vi "MB Serial Master Query.vi"(4 "Timeout":u32=10000, 6 "Serial Parameters":T1 {"Slave Address" format="%.0x"}, 8 "error in (no error)":errorcluster, 10 "Modbus Command":T2={"Function Code"=1, "Starting Address"=0, "Quantity"=0, "Data"=[], "Discrete"=[], "Index of Tags"=[]} {"Function Code" items=["Read Coils"=1, "Read Discrete Inputs"=2, "Read Holding Registers"=3, "Read Input Registers"=4, "Write Single Coil"=5, "Write Single Register"=6, "Read Exception Status"=7, "Write Multiple Coils"=15, "Write Multiple Registers"=16]}, 11 "VISA resource name":refnum<visa-resource-name>) -> (0 "error out":errorcluster, 1 "Exception Code":u8 format="%.0x", 2 "Registers":cluster{"Registers":u16[], "Discrete":bool[]}, 3 "VISA resource name out":refnum<visa-resource-name>, 5 "Modbus Data Unit Out":T3={"Function Code"=1, "Data"=[]} {"Function Code" items=["Read Coils"=1, "Read Discrete Inputs"=2, "Read Holding Registers"=3, "Read Input Registers"=4, "Write Single Coil"=5, "Write Single Register"=6, "Read Exception Status"=7, "Write Multiple Coils"=15, "Write Multiple Registers"=16]; "Data" format="%.0x"}, 7 "read buffer":string)   [LabVIEW 2020, in "ModBus Serial Master.lvlib"]
uses:
  ModBus Serial Master.lvlib
  MB Modbus Data Unit.ctl
  DriverCommon/MB Modbus Command.ctl
  DriverCommon.lvlib
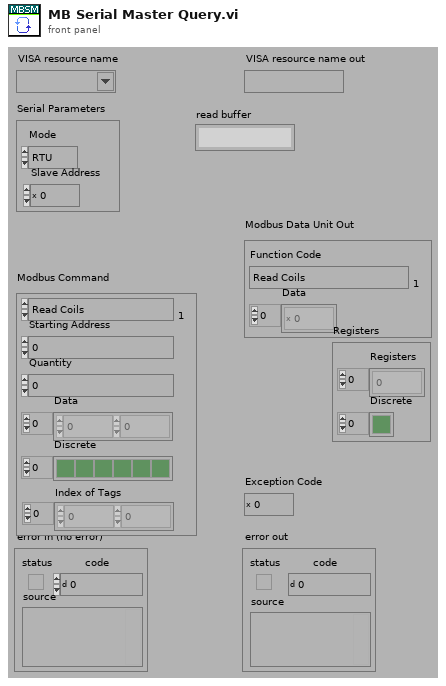
[diagram p1: front panel]
types:
  T1 = cluster{"Mode":enum16{"RTU", "ASCII"}, "Slave Address":u8}
  T2 = typedef "DriverCommon.lvlib/MB Modbus Command.ctl" = cluster{"Function Code":u8, "Starting Address":u16, "Quantity":u16, "Data":u16[], "Discrete":bool[], "Index of Tags":i32[]}
  T3 = typedef "ModBus Serial Master.lvlib/MB Modbus Data Unit.ctl" = cluster{"Function Code":u8, "Data":u8[]}
  T4 = typedef "DriverCommon.lvlib/MB Modbus Data Unit.ctl" = cluster{"Function Code":u8, "Data":u8[]}
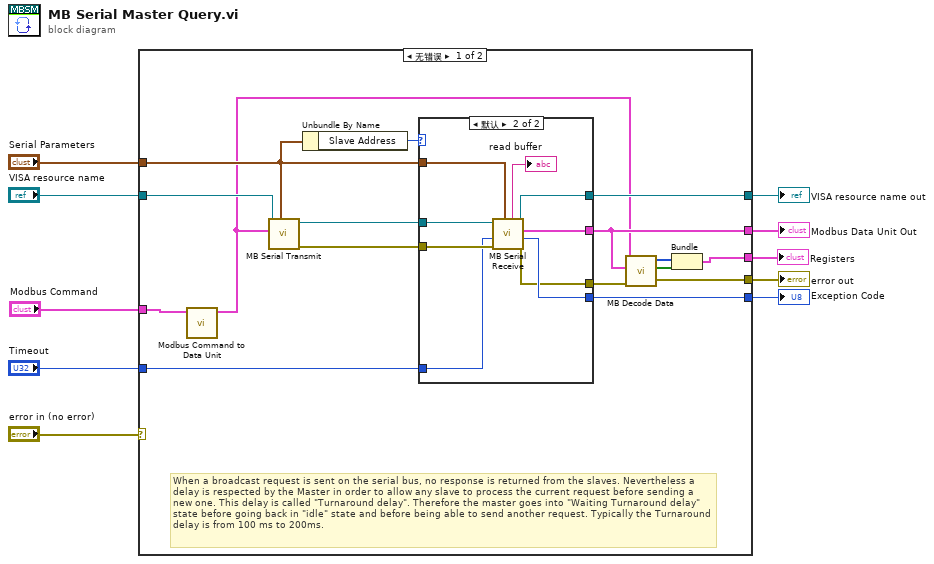
[diagram p0: block diagram]
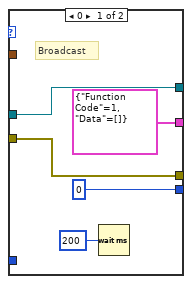
[diagram p2: hidden frame]
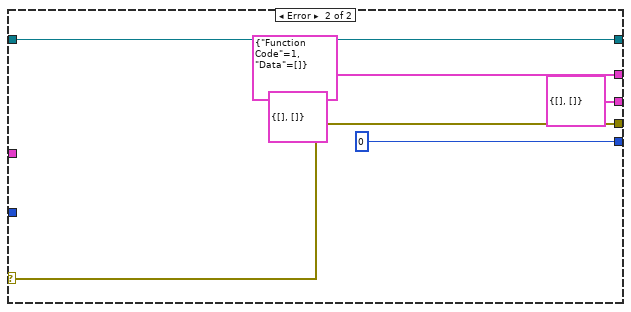
[diagram p3: hidden frame]
diagram:
  n1 = case shown="无错误" "error in (no error)" {
    selector: "error in (no error)" -> [_ w42]
    tunnel: [w22 T3 {"Function Code"=1, "Data"=[]} ("MODBUS Data Unit")] -> w5
    tunnel: [w23 u8 0 ("Exception Code")] -> w10
    tunnel: [w21 w42] -> w4
    tunnel: "VISA resource name" -> [w26 w45]
    tunnel: "Timeout" -> [w25 _]
    tunnel: [w24 w45] -> w7
    tunnel: "Modbus Command" -> [w14 _]
    tunnel: "Serial Parameters" -> [w16 _]
    tunnel: [w12 cluster{"Registers":u16[], "Discrete":bool[]} {"Registers"=[], "Discrete"=[]}] -> w1
    frame No Error {
      # "When a broadcast request is sent on the serial bus, no response is returned from the slaves. Nevertheless a delay is respected by the Master in order to allow any slave to process the current request before sending a new one. This delay is called \"Turnaround delay\". Therefore the master goes into \"Waiting Turnaround delay\" state before going back in \"idle\" state and before being able to send another request. Typically the Turnaround delay is from 100 ms to 200ms."
      n2 = call "Modbus Command to Data Unit.vi"("Modbus Command"=w14) -> ("Modbus Data Unit"=w15:T4)  [unwired: 10 in]
      n3 = call "MB Serial Transmit.vi"("Serial Parameters"=w16, "Modbus Data Unit"=w15, "VISA resource name"=w26) -> ("error out"=w19:errorcluster, "VISA resource name out"=w20:refnum<visa-resource-name>)  [unwired: 3 in, 4 out]
      n4 = Unbundle By Name(w16) -> ("Slave Address"=w18:u8)
      n5 = case shown="默认" w18 {
        tunnel: w20 -> [w31 w40]
        tunnel: w19 -> [w28 w39]
        tunnel: w25 -> [_ w38]
        tunnel: w16 -> [_ w37]
        tunnel: [w31 w36] -> w24
        tunnel: [u8 0 ("Exception Code") w35] -> w23
        tunnel: [T3 {"Function Code"=1, "Data"=[]} ("MODBUS Data Unit") w34] -> w22
        tunnel: [w28 w33] -> w17
        frame 0 {
          # "Broadcast"
          n6 = Wait (ms)(milliseconds to wait=u32 200) -> ()  [unwired: 1 out]
        }
        frame Default {
          n7 = call "MB Serial Receive.vi"("Serial Parameters"=w37, "error in (no error)"=w39, "Timeout"=w38, "VISA resource name"=w40) -> ("error out"=w33:errorcluster, "Exception Code"=w35:u8, "Modbus Data Unit"=w34:T4, "VISA resource name out"=w36:refnum<visa-resource-name>, "read buffer"=→"read buffer":string)  [unwired: 1 in, 2 out]
        }
      }
      n8 = call "MB Decode Data.vi"("error in (no error)"=w17, "Response MDU"=w22, "Request MDU"=w15) -> ("error out"=w21:errorcluster, "Discrete"=w11:bool[], "Registers"=w13:u16[])  [unwired: 6 in]
      n9 = Bundle("Registers"=w13, "Discrete"=w11) -> (w12:cluster{"Registers":u16[], "Discrete":bool[]})  [unwired: 1 out]
    }
    frame Error {
      (unwired) cluster{"Registers":u16[], "Discrete":bool[]} {"Registers"=[], "Discrete"=[]}
    }
  }
  "error out" <- w4
  "Exception Code" <- w10
  "VISA resource name out" <- w7
  "Modbus Data Unit Out" <- w5
  "Registers" <- w1
